vi "test Deploy Disabled Custom Device.vi"(8 "error in":errorcluster, 11 "TestCase in":refnum<class "Deployment.lvclass">) -> (0 "error out":errorcluster, 3 "TestCase out":refnum<class "Deployment.lvclass">)   [LabVIEW 2020, in "Deployment.lvclass"]
uses:
  Deployment.lvclass
  <vilib>/addons/_JKI Toolkits/VI Tester/TestCase.llb/TestCase.lvclass
  315b1c3a-44c8-49e8-b756-01f865c29b4a.vi
  <vilib>/NI/VeriStand Custom Device Testing Tools/VeriStandTestUtilities/VeriStandTestUtilities.lvlib
  Scripting/Ballard MIL-STD-1553 Scripting.lvlib
  C:/Users/nitest/Desktop/Git 2020/niveristand-custom-device-testing-tools/VeriStandTestCase/VeriStandTestCase.lvclass
  C:/Program Files (x86)/National Instruments/LabVIEW 2020/vi.lib/addons/_JKI Toolkits/VI Tester/TestCase.llb/TestCase.lvclass
  C:/Users/nitest/Desktop/Git 2020/niveristand-ballard-milStd1553-custom-device/Source/Custom Device Support/Tests/System/Deployment/Deployment.lvclass
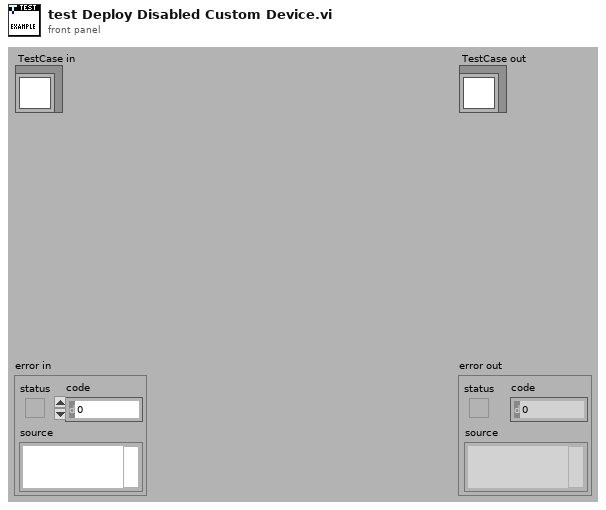
[diagram p1: front panel]
types:
  T1 = typedef "Custom Device API.lvlib/Custom Device Item Ref.ctl" = u64
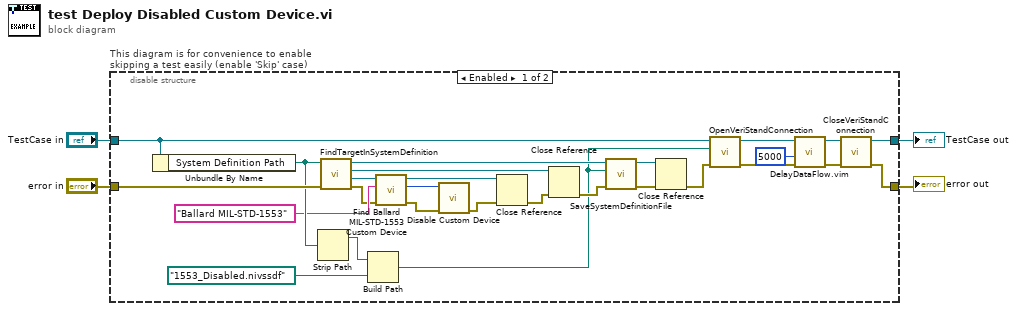
[diagram p0: block diagram]
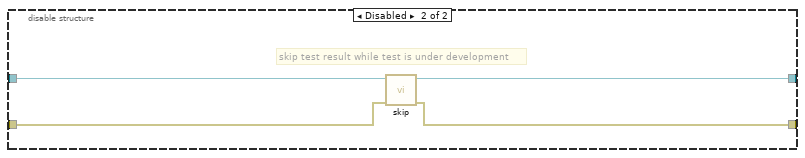
[diagram p2: hidden frame]
diagram:
  n1 = disable-structure "This diagram is for convenience to enable skipping a test easily (enable 'Skip' case)" shown="Enabled" {
    disable-tunnel: "TestCase in" -> [w24 w34]
    disable-tunnel: [w25 w32] -> w1
    disable-tunnel: [w27 w33] -> w3
    disable-tunnel: "error in" -> [w23 w31]
    frame Enabled {
      n2 = Unbundle By Name(w24) -> ("System Definition Path"=w21:path)
      n3 = Strip Path(path=w21) -> (stripped path=w6:path)  [unwired: 1 out]
      n4 = call <vilib>:"FindTargetInSystemDefinition.vi"("error in"=w23, "system definition path"=w21) -> ("error out"=w10:errorcluster, "Target"=w13:refnum<k24>, "Root"=w16:refnum<k24>, "System Definition"=w22:refnum<k24>)  [unwired: 6 in]
      n5 = Build Path(base path=w6, name or relative path=path "1553_Disabled.nivssdf") -> (appended path=w7:path)
      n6 = call "Find Ballard MIL-STD-1553 Custom Device.vi"("error in"=w10, "name"="Ballard MIL-STD-1553", "target in"=w13) -> ("error out"=w8:errorcluster, "Ballard MIL-STD 1553 custom device"=w9:T1, "target out"=w11:refnum<k24>)  [unwired: 5 in, 1 out]
      n7 = call "Disable Custom Device.vi"("error in"=w8, "Ballard MIL-STD 1553 custom device in"=w9) -> ("error out"=w5:errorcluster)  [unwired: 8 in, 1 out]
      n8 = Close Reference(reference=w11, error in (no error)=w5) -> (error out=w14:errorcluster)
      n9 = Close Reference(reference=w16, error in (no error)=w14) -> (error out=w15:errorcluster)
      n10 = call <vilib>:"SaveSystemDefinitionFile.vi"("error in (no error)"=w15, "System Definition File in"=w7, "System Definition Reference in"=w22) -> ("error out"=w18:errorcluster, "System Definition Reference out"=w19:refnum<k24>)  [unwired: 7 in]
      n11 = Close Reference(reference=w19, error in (no error)=w18) -> (error out=w17:errorcluster)
      n12 = call-dynamic "OpenVeriStandConnection.vi"("error in (no error)"=w17, "System Definition File"=w7, "VeriStand Test Case in"=w24) -> ("error out"=w30:errorcluster, "VeriStand Test Case out"=w26:refnum<class "Deployment.lvclass">)  [unwired: 6 in, 1 out]
      n13 = call "DelayDataFlow.vim"("value in"=w30, "milliseconds to wait"=u32 5000) -> ("value out"=w28:errorcluster)  [unwired: 2 in, 1 out]
      n14 = call-dynamic "CloseVeriStandConnection.vi"("error in (no error)"=w28, "VeriStand Test Case in"=w26) -> ("error out"=w27:errorcluster, "VeriStand Test Case out"=w25:refnum<class "Deployment.lvclass">)  [unwired: 8 in]
    }
    frame Disabled {
      # "skip test result while test is under development"
      n15 = call <vilib>:"skip.vi"("error in (no error)"=w31, "TestCase in"=w34) -> ("error out"=w33:errorcluster, "TestCase out"=w32:refnum<class "Deployment.lvclass">)  [unwired: 8 in]
    }
  }
  "error out" <- w3
  "TestCase out" <- w1
